vi "Parse Numeric.vi"(8 "error in (no error)":errorcluster, 10 "Index In":i32, 11 "JSON String":string) -> (0 "error out":errorcluster, 2 "Index Out":i32, 3 "JSON Value out":refnum<class "JSON Value.lvclass">)   [LabVIEW 2016, in "JSON Value.lvclass"]
uses:
  JSON Value.lvclass
  subVIs/Errors.ctl
  New JSON Value/New JSON (Numeric).vi
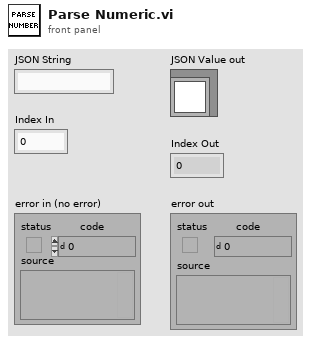
[diagram p1: front panel]
types:
  T1 = typedef "JSON Value.lvclass/Errors.ctl" = enum16{"No key", "Key path type", "Array OOB", "Type Mismatch", "Invalid Token"}
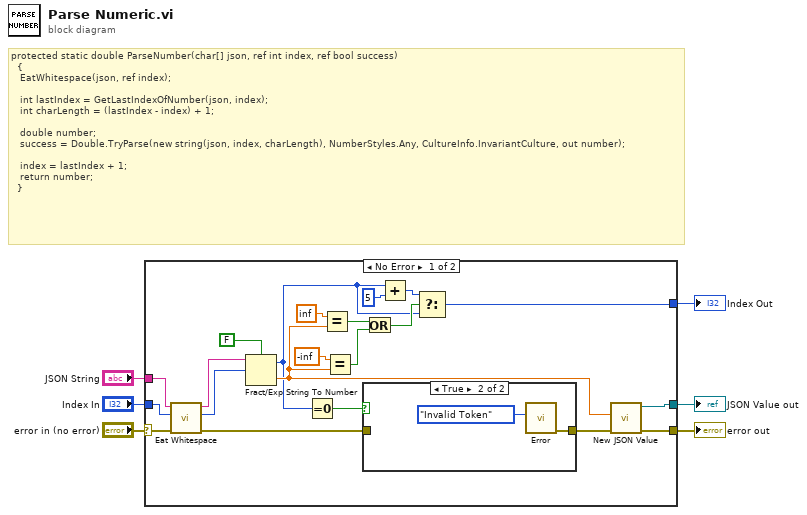
[diagram p0: block diagram]
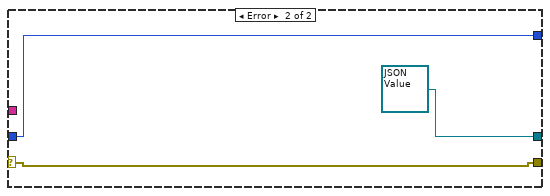
[diagram p3: hidden frame]
diagram:
  # "protected static double ParseNumber(char[] json, ref int index, ref bool success)\n\t\t{\n\t\t\tEatWhitespace(json, ref index);\n\n\t\t\tint lastIndex = GetLastIndexOfNumber(json, index);\n\t\t\tint charLength = (lastIndex - index) + 1;\n\n\t\t\tdouble number;\n\t\t\tsuccess = Double.TryParse(new string(json, index, charLength), NumberStyles.Any, CultureInfo.InvariantCulture, out number);\n\n\t\t\tindex = lastIndex + 1;\n\t\t\treturn number;\n\t\t}"
  n1 = case shown="No Error" "error in (no error)" {
    selector: "error in (no error)" -> [w26 w32]
    tunnel: [w23 w32] -> w5
    tunnel: [w22 refnum<class "JSON Value.lvclass"> refnum ("JSON out")] -> w1
    tunnel: "Index In" -> [w27 w33]
    tunnel: [w7 w33] -> w3
    tunnel: "JSON String" -> [w17 _]
    frame No Error {
      n2 = call "Eat Whitespace.vi"("error in (no error)"=w26, "Index In"=w27, "JSON String"=w17) -> ("error out"=w20:errorcluster, "Index Out"=w24:i32, "JSON String Passthrough"=w25:string)  [unwired: 6 in]
      n3 = Fract/Exp String To Number(use system decimal point (T)=FALSE, string=w25, offset=w24) -> (offset past number=w10:i32, number=w13:dbl)  [unwired: 1 in]
      n4 = Equal To 0?(x=w10) -> (x = 0?=w21:bool)
      n5 = Equal?(x=inf, y=w13) -> (x = y?=w15:bool)
      n6 = Equal?(x=-inf, y=w13) -> (x = y?=w12:bool)
      n7 = case shown="True" w21 {
        tunnel: w20 -> [w28 _]
        tunnel: [w28 w30] -> w19
        frame False {
        }
        frame True {
          n8 = call "Error.vi"(9:Errors."Invalid Token") -> ("error out"=w30:errorcluster)  [unwired: 9 in]
        }
      }
      n9 = Or(x=w15, y=w12) -> (x .or. y?=w11:bool)
      n10 = Add(x=w10, y=5) -> (x+y=w8:i32)
      n11 = Select(t=w8, s=w11, f=w10) -> (s? t:f=w7:i32)
      n12 = call-poly "New JSON Value.vi"("error in (no error)"=w19, "value"=w13) -> ("error out"=w23:errorcluster, "JSON Value out"=w22:refnum<class "JSON Value.lvclass">)  [unwired: 8 in]
    }
    frame Error {
    }
  }
  "error out" <- w5
  "Index Out" <- w3
  "JSON Value out" <- w1
